vi "SubVI_CoEIndexWrite.vi"(0 "Device address":string, 5 "Index":u16 format="%x", 7 "SubIndex":u8 format="%x", 9 "Data":u8[](array[numeric]), 11 "error in (no error)":errorcluster) -> (15 "error out":errorcluster)   [LabVIEW 2022 SP3, in "EtherCAT_Library.lvlib"]
uses:
  EtherCAT_Library.lvlib
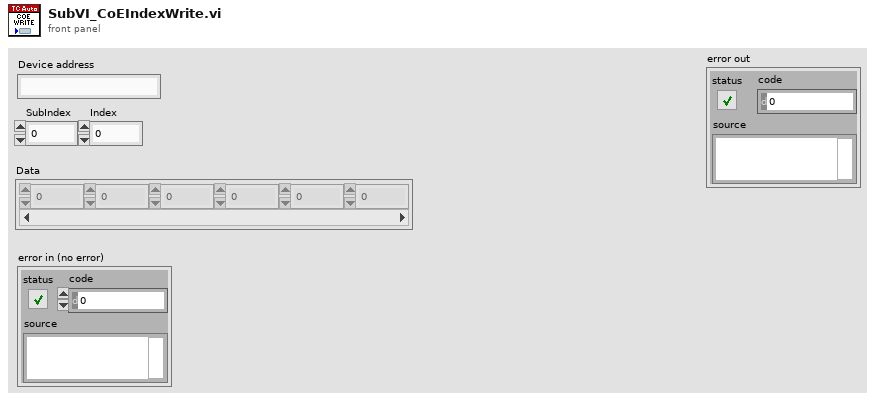
[diagram p1: front panel]
types:
  T1 = cluster{"Index":u16, "SubIndex":u8, "BitLength":u16, "ObjAccess":u16}
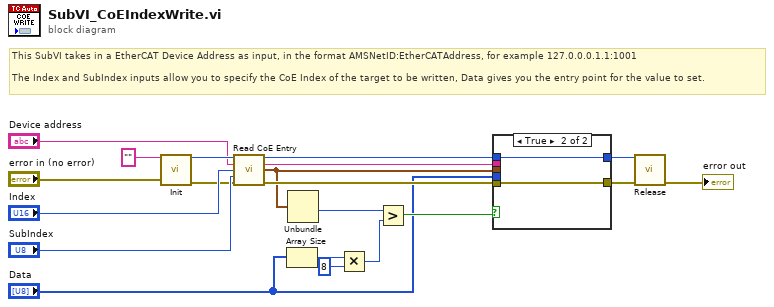
[diagram p0: block diagram]
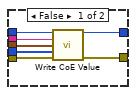
[diagram p2: hidden frame]
diagram:
  # "This SubVI takes in a EtherCAT Device Address as input, in the format AMSNetID:EtherCATAddress, for example 127.0.0.0.1.1:1001\n\nThe Index and SubIndex inputs allow you to specify the CoE Index of the target to be written, Data gives you the entry point for the value to set."
  n1 = call <userlib>:"Init.vi"("XMLDescription"="", "error in (no error)"="error in (no error)") -> ("Handle"=w17:u32, "error out"=w14:errorcluster)  [unwired: 9 in, 3 out]
  n2 = call <userlib>:"Read CoE Entry.vi"("Handle"=w17, "Device address"="Device address", "Index"="Index", "SubIndex"="SubIndex", "error in (no error)"=w14) -> ("Handle"=w12:u32, "Device address"=w11:string, "CoE Entry"=w7:T1, "error out"=w8:errorcluster)  [unwired: 6 in, 1 out]
  n3 = Array Size(array="Data") -> (size(s)=w3:i32)
  n4 = Unbundle(w7) -> ("BitLength"=w6:u16)  [unwired: 3 out]
  n5 = Multiply(x=w3, y=8) -> (x*y=w1:i32)
  n6 = Greater?(x=w6, y=w1) -> (0:w5:bool)
  n7 = case shown="True" w5 {
    tunnel: w12 -> [w27 w29]
    tunnel: w11 -> [w26 _]
    tunnel: [w21 w29] -> w10
    tunnel: [w22 w28] -> w9
    tunnel: w8 -> [w23 w28]
    tunnel: w7 -> [w25 _]
    tunnel: "Data" -> [w24 _]
    frame False {
      n8 = call <userlib>:"Write CoE Value.vi"("Handle"=w27, "Device address"=w26, "CoE entry"=w25, "Data"=w24, "error in (no error)"=w23) -> ("Handle"=w21:u32, "error out"=w22:errorcluster)  [unwired: 8 in, 1 out]
    }
    frame True {
    }
  }
  n9 = call <userlib>:"Release.vi"("Handle"=w10, "error in (no error)"=w9) -> ("error out"=→"error out":errorcluster)  [unwired: 13 in]
